vi "Get Release Status.vi"(8 "error in":errorcluster, 11 "Build Spec in":T1) -> (0 "error out":errorcluster, 3 "Build Spec out":T1, 4 "Is Release":bool)   [LabVIEW 2019, in "Project Sync Tools.lvclass"]
uses:
  Project Sync Tools.lvclass
  TypeDefs/BuildSpec Parameters.ctl
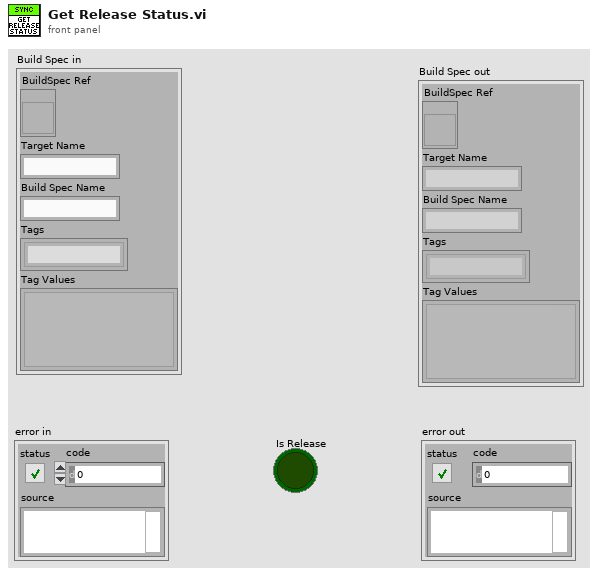
[diagram p1: front panel]
types:
  T1 = typedef "Project Sync Tools.lvclass/BuildSpec Parameters.ctl" = cluster{"BuildSpec Ref":refnum<vi>, "Target Name":string, "Build Spec Name":string, "Tags":string[], "Tag Values":variant[]}
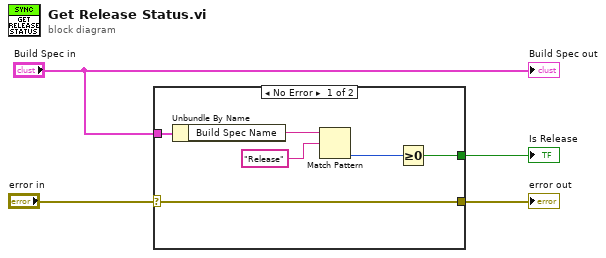
[diagram p0: block diagram]
diagram:
  n1 = case shown="No Error" "error in" {
    selector: "error in" -> [w5 w11]
    tunnel: "Build Spec in" -> [w10 _]
    tunnel: [w5 w11] -> w3
    tunnel: [w6 _] -> w1
    frame No Error {
      n2 = Unbundle By Name(w10) -> ("Build Spec Name"=w9:string)
      n3 = Match Pattern(string=w9, regular expression="Release") -> (offset past match=w7:i32)  [unwired: 1 in, 3 out]
      n4 = Greater Or Equal To 0?(x=w7) -> (x >= 0?=w6:bool)
    }
    frame Error {
    }
  }
  "error out" <- w3
  "Is Release" <- w1
  "Build Spec out" <- "Build Spec in"
